vi "Evaluate Data Errors.vi"(0 "Overwrite Error":i32, 5 "Stream Error":i32, 11 "Sweeps Running":bool) -> (8 "Data Error":bool)   [LabVIEW 2013]
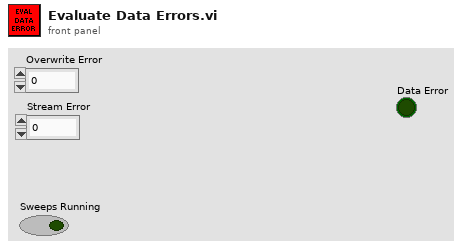
[diagram p1: front panel]
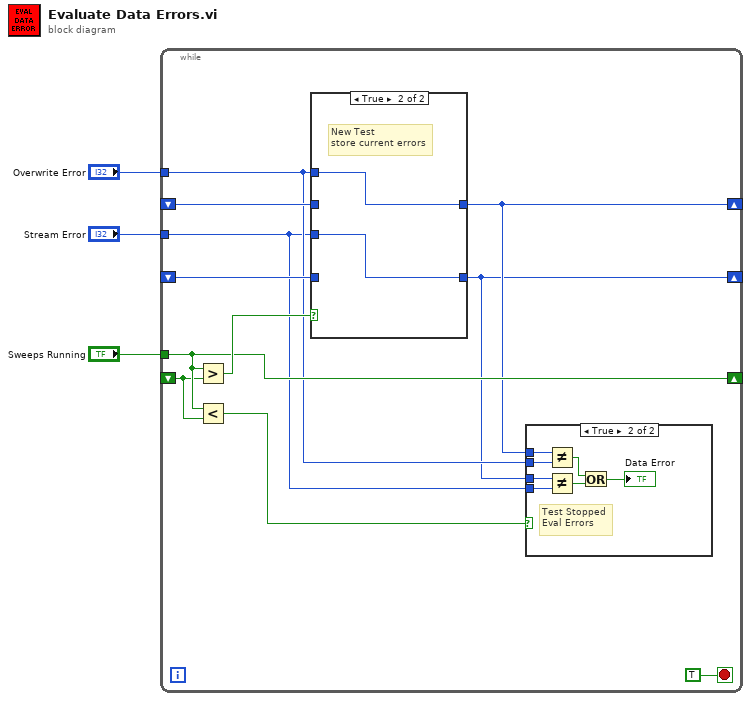
[diagram p0: block diagram]
diagram:
  n1 = while {
    tunnel: "Sweeps Running" -> [w10]
    tunnel: "Overwrite Error" -> [w6]
    tunnel: "Stream Error" -> [w4]
    shift-right: [w7] -> _
    shift-left: _ -> [w11]
    shift-right: [w5] -> _
    shift-left: _ -> [w12]
    shift-right: [w10] -> _
    shift-left: _ -> [w9]
    stop <- TRUE stop-if-true
    n2 = Greater?(x=w10, y=w9) -> (0:w13:bool)
    n3 = Less?(x=w10, y=w9) -> (x < y?=w8:bool)
    n4 = case shown="True" w13 {
      tunnel: w6 -> [_ w25]
      tunnel: w4 -> [_ w24]
      tunnel: [w23 w25] -> w7
      tunnel: [w22 w24] -> w5
      tunnel: w12 -> [w22 _]
      tunnel: w11 -> [w23 _]
      frame False {
      }
      frame True {
        # "New Test\nstore current errors"
      }
    }
    n5 = case shown="True" w8 {
      tunnel: w7 -> [_ w21]
      tunnel: w6 -> [_ w20]
      tunnel: w5 -> [_ w19]
      tunnel: w4 -> [_ w18]
      frame False {
      }
      frame True {
        # "Test Stopped\nEval Errors"
        n6 = Not Equal?(x=w21, y=w20) -> (x != y?=w16:bool)
        n7 = Not Equal?(x=w19, y=w18) -> (x != y?=w17:bool)
        n8 = Or(x=w16, y=w17) -> (x .or. y?=→"Data Error":bool)
      }
    }
  }
